vi "Nimbelink_Database_Ops_No_SQL_Open_Close.vi"(0 "Operation":T1(ring)=enum."Get Col Names", 1 "Record data":string[](array[string])=["wo12345", "123450001", "70B3D55A8100", "A1001234567890", "Joe", "2013-05-07 10:28:19", "100013", "353123456789012", "89123456789012345678", "612-555-1212", "Pass", "", "", "", "", "", "", "", "", "", "", "", "", "", "", "", "", "", "", "", "", "", "", "", "", "", "", "", "", "", "", "", "", "", "", "", "", "", "", "", "", "", "", "", "", "", "", "", "", "", "", "", "12:01:00"], 3 "Connection In":refnum<k7>, 4 "SQL Query":string="Insert into dbo.test_data VALUES ", 5 "Error in (no error)":errorcluster, 6 "Find column":u16(ring) items=["work_order", "btw_sn", "mac", "meid", "operator", "datetime", "part_number", "imei", "sim_id", "phone", "test_result"], 7 "Find data":string, 10 "table name":string="test_data", 11 "Insert fields":i32=39) -> (12 "Found?":bool, 13 "Last test passed?":bool, 14 "RecordSet":string[][](array[string]), 15 "Column Names":string[](array[string])=["work_order", "btw_sn", "mac", "meid", "operator", "date_time", "part_number", "imei", "sim_id", "phone_number", "test_result", "board_sn", "test_time", "test_program", "test_version", "extra1", "extra2", "guid", "extra3", "extra4", "extra5", "extra6", "extra7"], 16 "Connection Out":refnum<k7>, 17 "Find return string":string, 18 "Records":i32, 19 "Error out":errorcluster)   [LabVIEW 2013]
panel:
  out "Final query string":string="select column_name,* from information_schema.columns\n where table_name = 'test_data'\norder by ordinal_position"
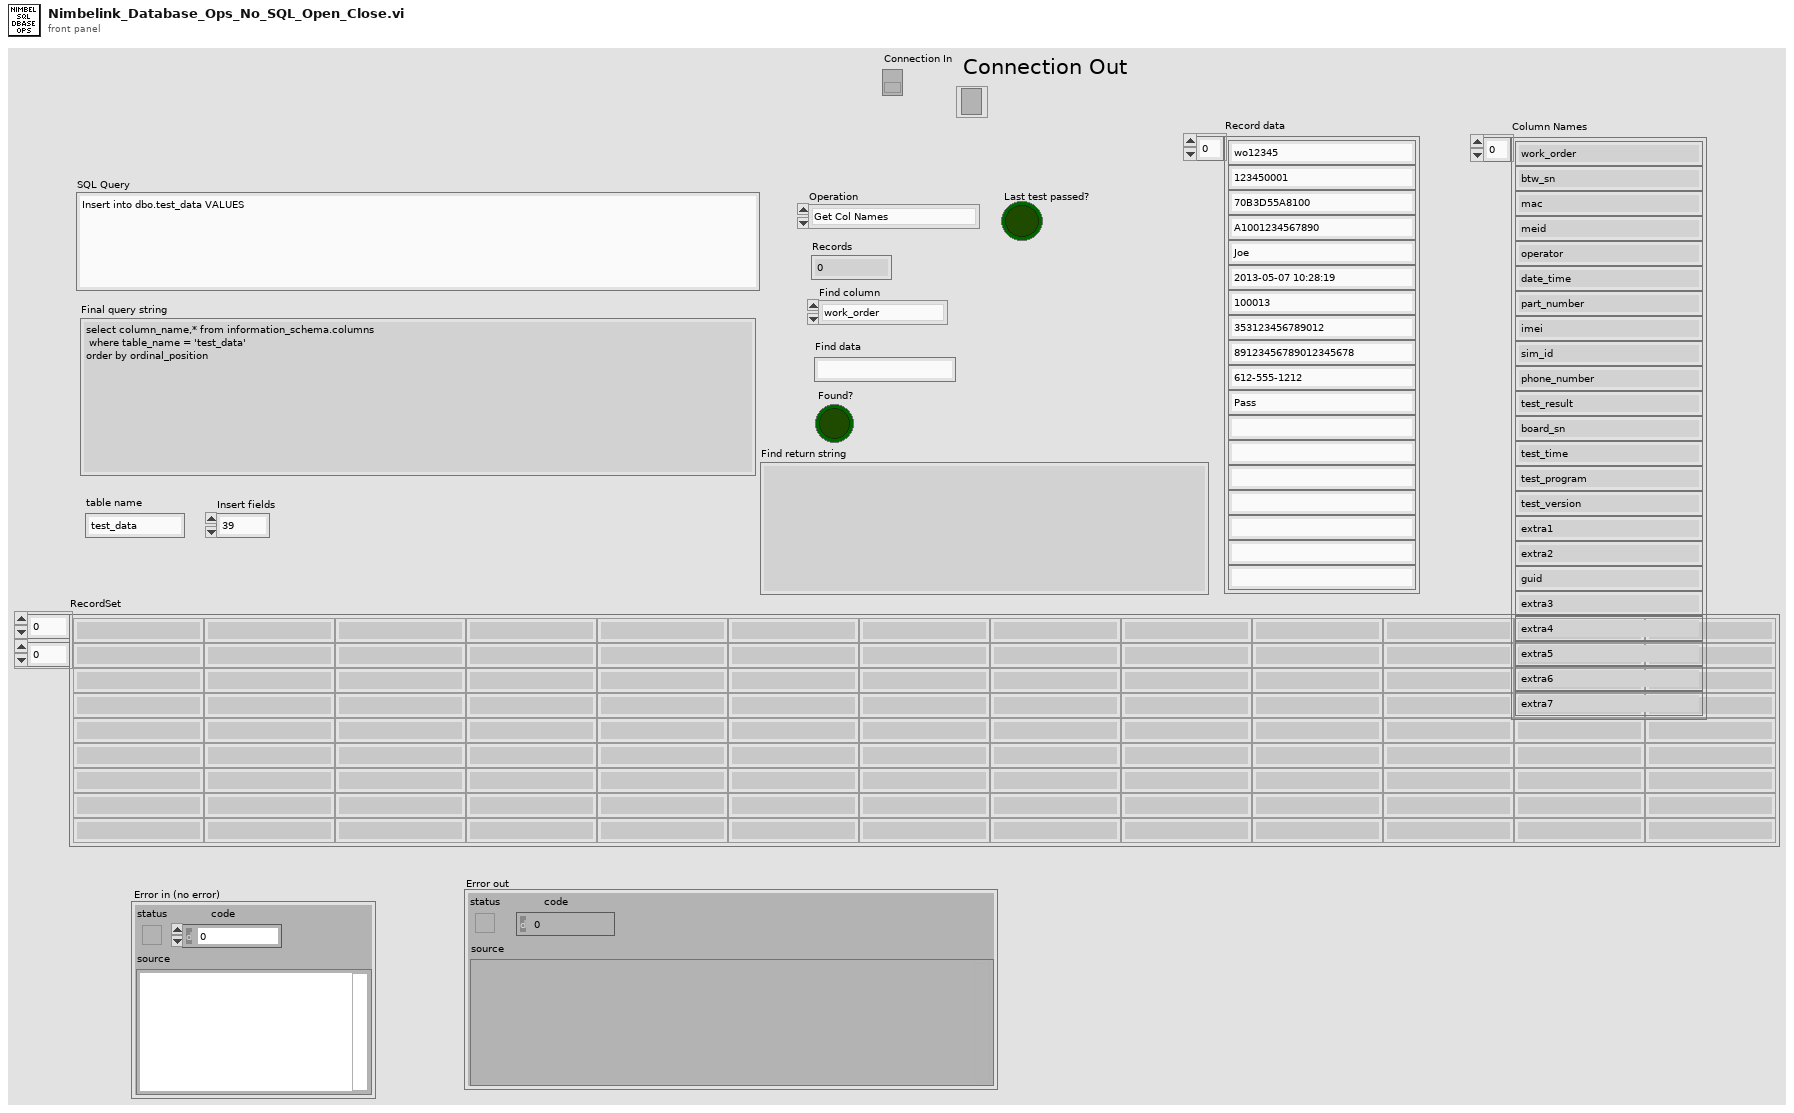
[diagram p1: front panel]
types:
  T1 = enum16{"Query", "Insert", "Select", "Dump Recs", "Get Rec Count", "Get Col Names", "Insert all fields", "Find", "Get last test result", "Get work order qty", "Set work order qty", "Save test report", "Get test report", "Execute query no data", "Select count", "Query and return row 0 col 0"}
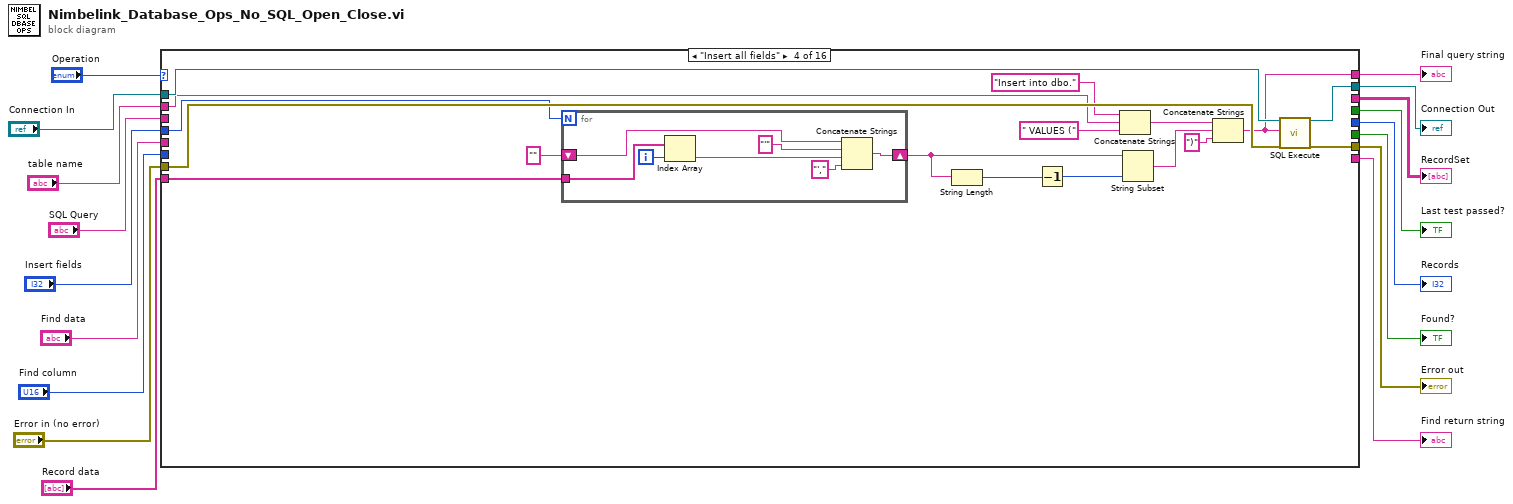
[diagram p0: block diagram]
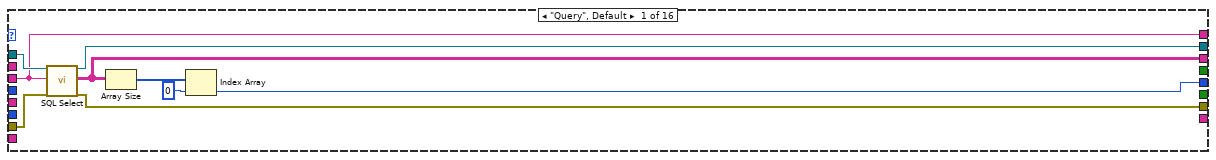
[diagram p2: hidden frame]
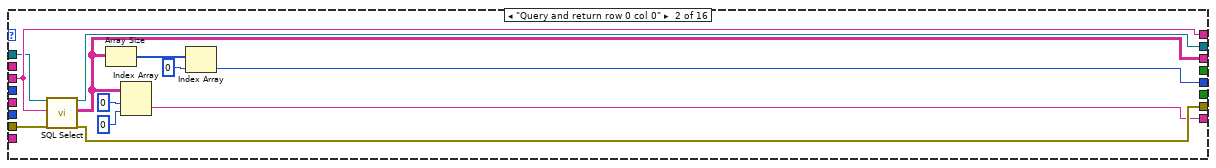
[diagram p3: hidden frame]
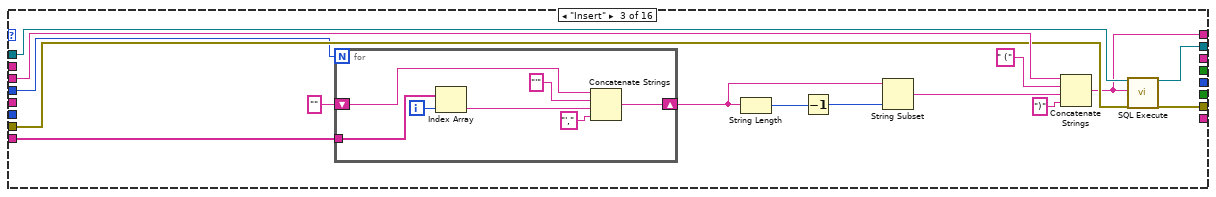
[diagram p4: hidden frame]
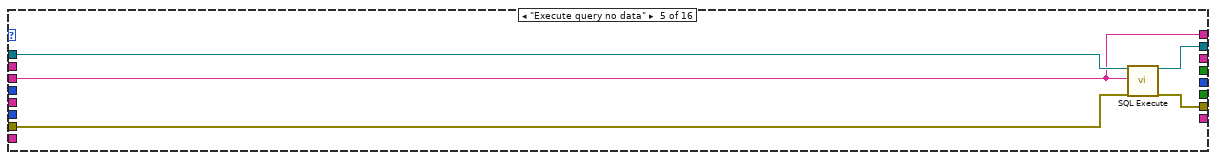
[diagram p5: hidden frame]
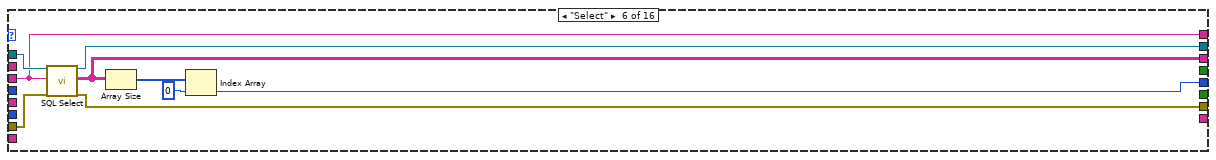
[diagram p6: hidden frame]
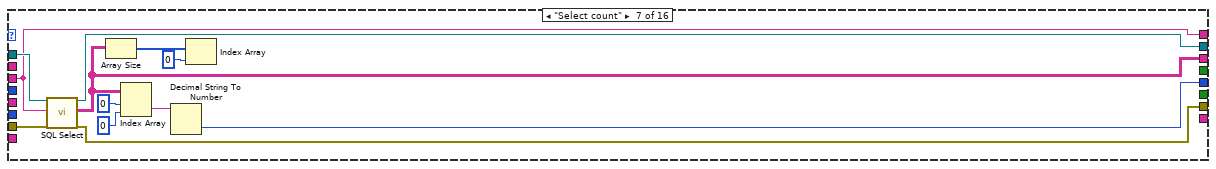
[diagram p7: hidden frame]
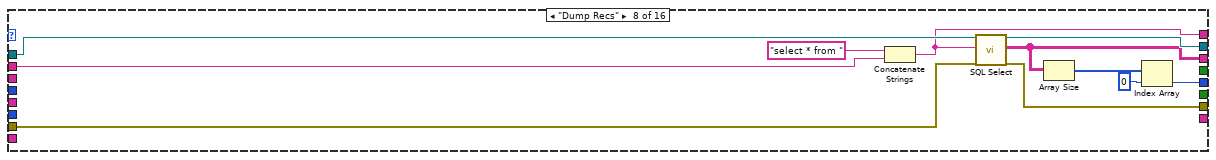
[diagram p8: hidden frame]
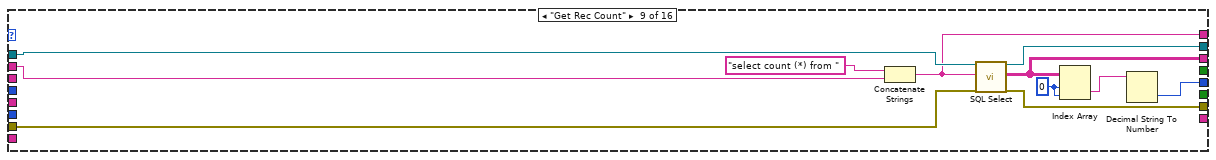
[diagram p9: hidden frame]
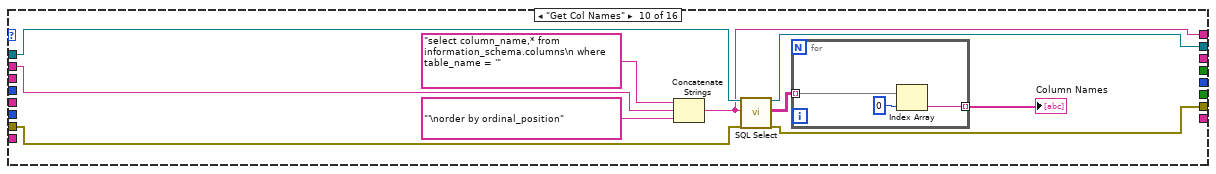
[diagram p10: hidden frame]
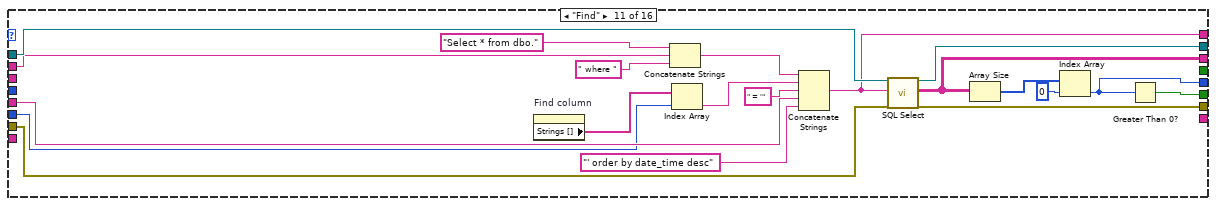
[diagram p11: hidden frame]
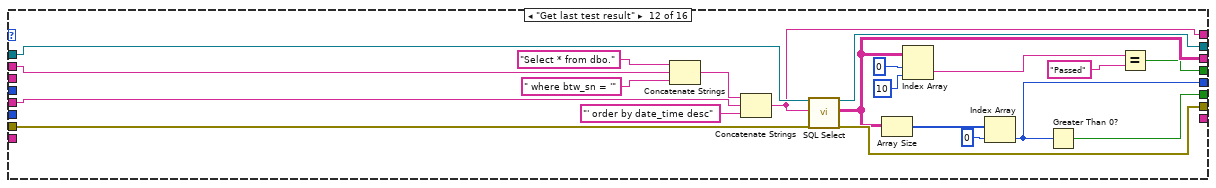
[diagram p12: hidden frame]
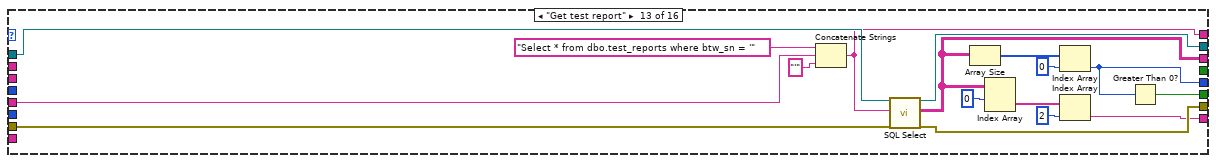
[diagram p13: hidden frame]
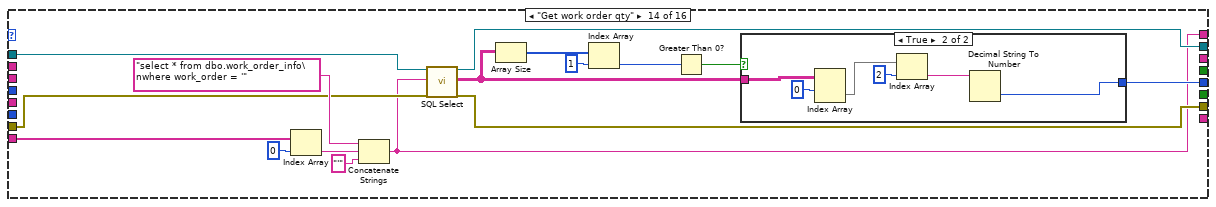
[diagram p14: hidden frame]
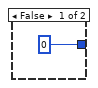
[diagram p15: hidden frame]
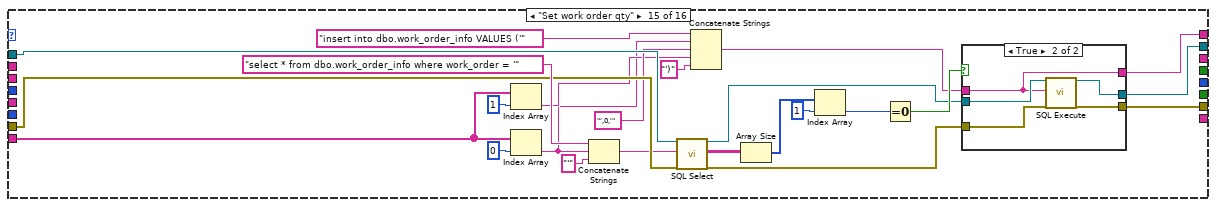
[diagram p16: hidden frame]
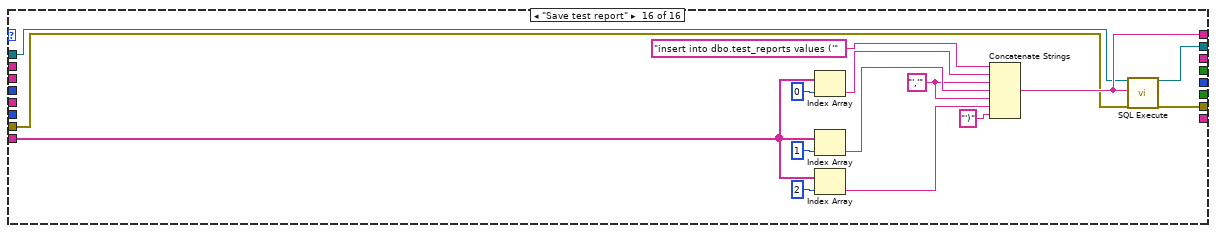
[diagram p18: hidden frame]
diagram:
  n1 = case shown="\"Insert all fields\"" "Operation" {
    tunnel: [w25 w37 w53 w61 w89 w95 w107 w118 w129 w138 w159 w183 w200 w208 w234 w268] -> w2
    tunnel: [w23 w29 w52 w62 w88 w96 w108 w119 w130 w137 w161 w185 w202 w210 w233 w267] -> w1
    tunnel: "Connection In" -> [w24 w30 w51 w77 w87 w97 w109 w121 w132 w142 w162 w186 w203 w211 w250 w264]
    tunnel: "Error in (no error)" -> [w26 w38 w41 w69 w86 w98 w110 w120 w131 w141 w160 w184 w201 w213 w247 w265]
    tunnel: "SQL Query" -> [w22 w36 w46 _ w85 w94 w106 _ _ _ _ _ _ _ _ _]
    tunnel: [w19 w32 _ _ _ w91 w102 w114 w124 _ w156 w171 w191 _ _ _] -> w13
    tunnel: "Record data" -> [_ _ w50 w76 _ _ _ _ _ _ _ _ _ w212 w239 w263]
    tunnel: [w22 w36 w40 w68 w85 w94 w106 w117 w126 w136 w155 w180 w197 w207 w232 w266] -> w14
    tunnel: "table name" -> [_ _ _ w67 _ _ _ w116 w127 w134 w152 w177 _ _ _ _]
    tunnel: [w18 w33 _ _ _ w90 w101 w111 w123 _ w149 w174 w195 w209 _ _] -> w11
    tunnel: [_ _ _ _ _ _ _ _ _ _ w148 w173 w194 _ _ _] -> w10
    tunnel: "Find data" -> [_ _ _ _ _ _ _ _ _ _ w147 w172 w193 _ _ _]
    tunnel: "Find column" -> [_ _ _ _ _ _ _ _ _ _ w146 _ _ _ _ _]
    tunnel: [_ _ _ _ _ _ _ _ _ _ _ w166 _ _ _ _] -> w7
    tunnel: "Insert fields" -> [_ _ w39 w63 _ _ _ _ _ _ _ _ _ _ _ _]
    tunnel: [_ w27 _ _ _ _ _ _ _ _ _ _ w188 _ _ _] -> w5
    frame "Query", Default {
      n2 = call "SQL Select.vi"("Connection In"=w24, "SQL Query"=w22, "Error in (no error)"=w26) -> ("Connection Out"=w23:refnum<k7>, "Data"=w19:string[][], "Error out"=w25:errorcluster)  [unwired: 14 in]
      n3 = Array Size(array=w19) -> (size(s)=w21:i32[])
      n4 = Index Array(array=w21, index=0) -> (element=w18:i32)
    }
    frame "Query and return row 0 col 0" {
      n5 = call "SQL Select.vi"("Connection In"=w30, "SQL Query"=w36, "Error in (no error)"=w38) -> ("Connection Out"=w29:refnum<k7>, "Data"=w32:string[][], "Error out"=w37:errorcluster)  [unwired: 14 in]
      n6 = Array Size(array=w32) -> (size(s)=w35:i32[])
      n7 = Index Array(array=w32, index (row)=0, index (col)=0 ("disabled index (col)")) -> (element=w27:string)
      n8 = Index Array(array=w35, index=0) -> (element=w33:i32)
    }
    frame "Insert" {
      n9 = for {
        N: w39 -> [_]
        tunnel: w50 -> [w56]
        shift-right: [w59] -> w43
        shift-left: "" -> [w58]
        i -> [w55]
        n10 = Index Array(array=w56, index=w55) -> (element=w54:string)
        n11 = Concatenate Strings(w58, "'" ("string"), w54, "'," ("string")) -> (w59:string)
      }
      n12 = String Length(string=w43) -> (length=w45:i32)
      n13 = Decrement(x=w45) -> (x-1=w44:i32)
      n14 = String Subset(string=w43, length (rest)=w44) -> (substring=w42:string)  [unwired: 1 in]
      n15 = Concatenate Strings(w46, " (" ("string"), w42, ")") -> (w40:string)
      n16 = call "SQL Execute.vi"("Connection In"=w51, "SQL Query"=w40, "Error in (no error)"=w41) -> ("Connection Out"=w52:refnum<k7>, "Error out"=w53:errorcluster)  [unwired: 15 in]
    }
    frame "Insert all fields" {
      n17 = for {
        N: w63 -> [_]
        tunnel: w76 -> [w80]
        shift-right: [w83] -> w71
        shift-left: "" -> [w82]
        i -> [w79]
        n18 = Index Array(array=w80, index=w79) -> (element=w78:string)
        n19 = Concatenate Strings(w82, "'" ("string"), w78, "'," ("string")) -> (w83:string)
      }
      n20 = String Length(string=w71) -> (length=w73:i32)
      n21 = Decrement(x=w73) -> (x-1=w72:i32)
      n22 = Concatenate Strings("Insert into dbo." ("string"), w67, " VALUES (" ("string")) -> (w66:string)
      n23 = String Subset(string=w71, length (rest)=w72) -> (substring=w70:string)  [unwired: 1 in]
      n24 = Concatenate Strings(w66, w70, ")") -> (w68:string)
      n25 = call "SQL Execute.vi"("Connection In"=w77, "SQL Query"=w68, "Error in (no error)"=w69) -> ("Connection Out"=w62:refnum<k7>, "Error out"=w61:errorcluster)  [unwired: 15 in]
    }
    frame "Execute query no data" {
      n26 = call "SQL Execute.vi"("Connection In"=w87, "SQL Query"=w85, "Error in (no error)"=w86) -> ("Connection Out"=w88:refnum<k7>, "Error out"=w89:errorcluster)  [unwired: 15 in]
    }
    frame "Select" {
      n27 = call "SQL Select.vi"("Connection In"=w97, "SQL Query"=w94, "Error in (no error)"=w98) -> ("Connection Out"=w96:refnum<k7>, "Data"=w91:string[][], "Error out"=w95:errorcluster)  [unwired: 14 in]
      n28 = Array Size(array=w91) -> (size(s)=w93:i32[])
      n29 = Index Array(array=w93, index=0) -> (element=w90:i32)
    }
    frame "Select count" {
      n30 = call "SQL Select.vi"("Connection In"=w109, "SQL Query"=w106, "Error in (no error)"=w110) -> ("Connection Out"=w108:refnum<k7>, "Data"=w102:string[][], "Error out"=w107:errorcluster)  [unwired: 14 in]
      n31 = Array Size(array=w102) -> (size(s)=w105:i32[])
      n32 = Index Array(array=w102, index (row)=0, index (col)=0 ("disabled index (col)")) -> (element=w99:string)
      n33 = Decimal String To Number(string=w99) -> (number=w101:i32)  [unwired: 2 in, 1 out]
      n34 = Index Array(array=w105, index=0) -> ()  [unwired: 1 out]
    }
    frame "Dump Recs" {
      n35 = Concatenate Strings("select * from " ("SQL Query"), w116) -> (w117:string)
      n36 = call "SQL Select.vi"("Connection In"=w121, "SQL Query"=w117, "Error in (no error)"=w120) -> ("Connection Out"=w119:refnum<k7>, "Data"=w114:string[][], "Error out"=w118:errorcluster)  [unwired: 14 in]
      n37 = Array Size(array=w114) -> (size(s)=w113:i32[])
      n38 = Index Array(array=w113, index=0) -> (element=w111:i32)
    }
    frame "Get Rec Count" {
      w128 = 0 ("index (row)")
      n39 = Concatenate Strings("select count (*) from " ("SQL Query"), w127) -> (w126:string)
      n40 = call "SQL Select.vi"("Connection In"=w132, "SQL Query"=w126, "Error in (no error)"=w131) -> ("Connection Out"=w130:refnum<k7>, "Data"=w124:string[][], "Error out"=w129:errorcluster)  [unwired: 14 in]
      n41 = Index Array(array=w124, index (row)=w128, index (col)=w128) -> (element=w122:string)
      n42 = Decimal String To Number(string=w122) -> (number=w123:i32)  [unwired: 2 in, 1 out]
    }
    frame "Get Col Names" {
      n43 = Concatenate Strings("select column_name,* from information_schema.columns\n where table_name = '" ("SQL Query"), w134, "'\norder by ordinal_position" ("SQL Query")) -> (w136:string)
      n44 = call "SQL Select.vi"("Connection In"=w142, "SQL Query"=w136, "Error in (no error)"=w141) -> ("Connection Out"=w137:refnum<k7>, "Data"=w140:string[][], "Error out"=w138:errorcluster)  [unwired: 14 in]
      n45 = for {
        tunnel: w140 -> [w145] mode=indexing
        tunnel: [w144] -> w139 mode=indexing
        n46 = Index Array(array=w145, index=0 ("index (col)")) -> (element=w144:string)
      }
      "Column Names" <- w139
    }
    frame "Find" {
      n47 = property on="Find column" class="Ring (strict)"() -> ("Strings []"=w165:string[])  [unwired: 2 in, 2 out]
      n48 = Concatenate Strings("Select * from dbo." ("string"), w152, " where " ("string")) -> (w154:string)
      n49 = Index Array(array=w165, index=w146) -> (element=w164:string)
      n50 = Concatenate Strings(w154, w164, " = '" ("string"), w147, "' order by date_time desc" ("string")) -> (w155:string)
      n51 = call "SQL Select.vi"("Connection In"=w162, "SQL Query"=w155, "Error in (no error)"=w160) -> ("Connection Out"=w161:refnum<k7>, "Data"=w156:string[][], "Error out"=w159:errorcluster)  [unwired: 14 in]
      n52 = Array Size(array=w156) -> (size(s)=w157:i32[])
      n53 = Index Array(array=w157, index=0) -> (element=w149:i32)
      n54 = Greater Than 0?(x=w149) -> (x > 0?=w148:bool)
    }
    frame "Get last test result" {
      n55 = Concatenate Strings("Select * from dbo." ("string"), w177, " where btw_sn = '" ("string")) -> (w179:string)
      n56 = Concatenate Strings(w179, w172, "' order by date_time desc" ("string")) -> (w180:string)
      n57 = call "SQL Select.vi"("Connection In"=w186, "SQL Query"=w180, "Error in (no error)"=w184) -> ("Connection Out"=w185:refnum<k7>, "Data"=w171:string[][], "Error out"=w183:errorcluster)  [unwired: 14 in]
      n58 = Array Size(array=w171) -> (size(s)=w181:i32[])
      n59 = Index Array(array=w171, index (row)=0, index (col)=10 ("disabled index (col)")) -> (element=w168:string)
      n60 = Index Array(array=w181, index=0) -> (element=w174:i32)
      n61 = Greater Than 0?(x=w174) -> (x > 0?=w173:bool)
      n62 = Equal?(x=w168, y="Passed") -> (x = y?=w166:bool)
    }
    frame "Get test report" {
      n63 = Concatenate Strings("Select * from dbo.test_reports where btw_sn = '" ("string"), w193, "'" ("string")) -> (w197:string)
      n64 = call "SQL Select.vi"("Connection In"=w203, "SQL Query"=w197, "Error in (no error)"=w201) -> ("Connection Out"=w202:refnum<k7>, "Data"=w191:string[][], "Error out"=w200:errorcluster)  [unwired: 14 in]
      n65 = Array Size(array=w191) -> (size(s)=w198:i32[])
      n66 = Index Array(array=w191, index (row)=0) -> (element=w189:string[])  [unwired: 1 in]
      n67 = Index Array(array=w198, index=0) -> (element=w195:i32)
      n68 = Index Array(array=w189, index=2) -> (element=w188:string)
      n69 = Greater Than 0?(x=w195) -> (x > 0?=w194:bool)
    }
    frame "Get work order qty" {
      n70 = Index Array(array=w212, index=0) -> (element=w215:string)
      n71 = Concatenate Strings("select * from dbo.work_order_info\nwhere work_order = '" ("SQL Query"), w215, "'" ("string")) -> (w207:string)
      n72 = call "SQL Select.vi"("Connection In"=w211, "SQL Query"=w207, "Error in (no error)"=w213) -> ("Connection Out"=w210:refnum<k7>, "Data"=w206:string[][], "Error out"=w208:errorcluster)  [unwired: 14 in]
      n73 = Array Size(array=w206) -> (size(s)=w205:i32[])
      n74 = Index Array(array=w205, index=1) -> (element=w204:i32)
      n75 = Greater Than 0?(x=w204) -> (x > 0?=w214:bool)
      n76 = case shown="True" w214 {
        tunnel: w206 -> [_ w225]
        tunnel: [0 w224] -> w209
        frame False {
        }
        frame True {
          n77 = Index Array(array=w225, index (row)=0 ("index")) -> (element=w223:string[])  [unwired: 1 in]
          n78 = Index Array(array=w223, index=2) -> (element=w221:string)
          n79 = Decimal String To Number(string=w221) -> (number=w224:i32)  [unwired: 2 in, 1 out]
        }
      }
    }
    frame "Set work order qty" {
      n80 = Index Array(array=w239, index=1) -> (element=w240:string)
      n81 = Index Array(array=w239, index=0) -> (element=w238:string)
      n82 = Concatenate Strings("select * from dbo.work_order_info where work_order = '" ("SQL Query"), w238, "'" ("string")) -> (w231:string)
      n83 = call "SQL Select.vi"("Connection In"=w250, "SQL Query"=w231, "Error in (no error)"=w247) -> ("Connection Out"=w236:refnum<k7>, "Data"=w227:string[][], "Error out"=w235:errorcluster)  [unwired: 14 in]
      n84 = Concatenate Strings("insert into dbo.work_order_info VALUES ('" ("SQL Query"), w238, "',0,'" ("string"), w240, "')" ("string")) -> (w228:string)
      n85 = Array Size(array=w227) -> (size(s)=w230:i32[])
      n86 = Index Array(array=w230, index=1) -> (element=w229:i32)
      n87 = Equal To 0?(x=w229) -> (x = 0?=w245:bool)
      n88 = case shown="True" w245 {
        tunnel: w236 -> [w252 w255]
        tunnel: w228 -> [w251 w254]
        tunnel: w235 -> [w253 w258]
        tunnel: [w253 w257] -> w234
        tunnel: [w252 w256] -> w233
        tunnel: [w251 w254] -> w232
        frame False {
        }
        frame True {
          n89 = call "SQL Execute.vi"("Connection In"=w255, "SQL Query"=w254, "Error in (no error)"=w258) -> ("Connection Out"=w256:refnum<k7>, "Error out"=w257:errorcluster)  [unwired: 15 in]
        }
      }
    }
    frame "Save test report" {
      w261 = "','" ("string")
      n90 = Index Array(array=w263, index=0) -> (element=w269:string)
      n91 = Index Array(array=w263, index=1) -> (element=w270:string)
      n92 = Index Array(array=w263, index=2) -> (element=w260:string)
      n93 = Concatenate Strings("insert into dbo.test_reports values ('" ("SQL Query"), w269, w261, w270, w261, w260, "')" ("string")) -> (w266:string)
      n94 = call "SQL Execute.vi"("Connection In"=w264, "SQL Query"=w266, "Error in (no error)"=w265) -> ("Connection Out"=w267:refnum<k7>, "Error out"=w268:errorcluster)  [unwired: 15 in]
    }
  }
  "Error out" <- w2
  "RecordSet" <- w13
  "Final query string" <- w14
  "Records" <- w11
  "Found?" <- w10
  "Last test passed?" <- w7
  "Find return string" <- w5
  "Connection Out" <- w1
